vi "COMI US Change Sample Freq.vi"(10 "dwSampleFreq":u32, 11 "hDevice":u32) -> (3 "hDevice out":u32)   [LabVIEW 2017, in "Comidll.lvlib"]
doc: "void (COMI_US_ChangeSampleFreq) (HANDLE hDevice, unsigned long dwSampleFreq);"
uses:
  <userlib>/Comidll/Comidll.lvlib
  <userlib>/Comidll/Comidll.dll
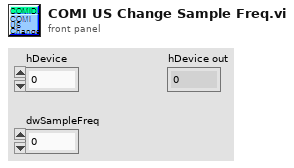
[diagram p1: front panel]
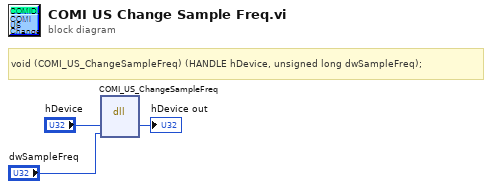
[diagram p0: block diagram]
diagram:
  # "void\t(COMI_US_ChangeSampleFreq) (HANDLE hDevice, unsigned long dwSampleFreq);"
  n1 = dll-call lib="C:/Program Files/National Instruments/LabVIEW 2017/user.lib/Comidll/Comidll.*" fn="COMI_US_ChangeSampleFreq"("hDevice"="hDevice", "dwSampleFreq"="dwSampleFreq") -> ("hDevice"=→"hDevice out":u32)  [unwired: 5 in, 2 out]
